vi "Get Module Identifier.vi"(8 "error in (no error)":errorcluster, 10 "Module path":string, 11 "Routing and Faulting BaseNodeType in":refnum<k24>) -> (0 "error out":errorcluster, 1 "Found?":bool, 2 "Module identifier":string, 3 "Routing and Faulting BaseNodeType out":refnum<k24>)   [LabVIEW 2017, in "Routing and Faulting Scripting.lvlib"]
uses:
  Routing and Faulting Scripting.lvlib
  NationalInstruments.VeriStand.SystemStorage
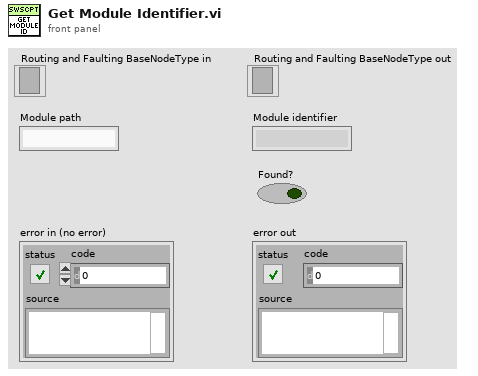
[diagram p1: front panel]
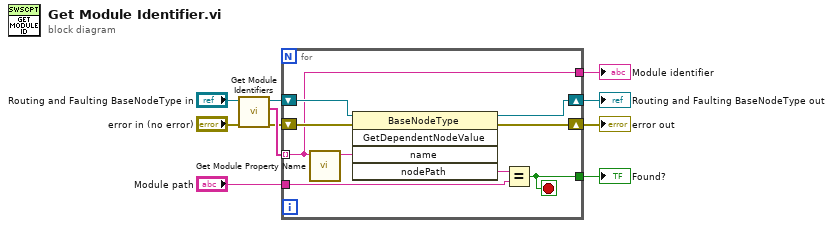
[diagram p0: block diagram]
diagram:
  n1 = call "Get Module Identifiers.vi"("error in (no error)"="error in (no error)", ".NET Refnum in"="Routing and Faulting BaseNodeType in") -> ("error out"=w1:errorcluster, "Module Identifier"=w7:string[], ".NET Refnum out"=w2:refnum<k24>)  [unwired: 7 in]
  n2 = for {
    tunnel: w7 -> [w11] mode=indexing
    tunnel: "Module path" -> [w12]
    tunnel: [w11] -> w8
    shift-right: [w16] -> w4
    shift-left: w1 -> [w19]
    tunnel: [w15] -> w3
    shift-right: [w14] -> w5
    shift-left: w2 -> [w18]
    stop <- w15 stop-if-true
    n3 = call "Get Module Property Name.vi"("Module ID"=w11) -> ("Module Property Name"=w13:string)  [unwired: 10 in]
    n4 = invoke class="BaseNodeType" method="GetDependentNodeValue"(reference=w18, error in=w19, "name"=w13) -> (reference out=w14:refnum<k24>, error out=w16:errorcluster, "nodePath"=w17:string)  [unwired: 2 in, 2 out]
    n5 = Equal?(x=w17, y=w12) -> (x = y?=w15:bool)
  }
  "Module identifier" <- w8
  "Routing and Faulting BaseNodeType out" <- w5
  "error out" <- w4
  "Found?" <- w3
